vi "Rampfunction (SubVI).vi"(0 "Time":dbl, 1 "Ramp activate":bool, 5 "Ramp td [s]":dbl=1.0, 7 "Ramp tr [s]":dbl=2.0, 9 "Ramp t_ramp [s]":dbl=20.0, 11 "Ramp ymax":dbl=3.5, 12 "Direction":bool) -> (4 "y":dbl, 6 "ramp time":dbl, 8 "Ramp array":dbl[][](array[numeric]), 10 "Ramp active":bool, 15 "Ramp done":bool)   [LabVIEW 2017]
uses:
  <vilib>/gmath/NI_Gmath.lvlib
panel:
  out "y array":dbl[](array[numeric])
  out "time array":dbl[](array[numeric])
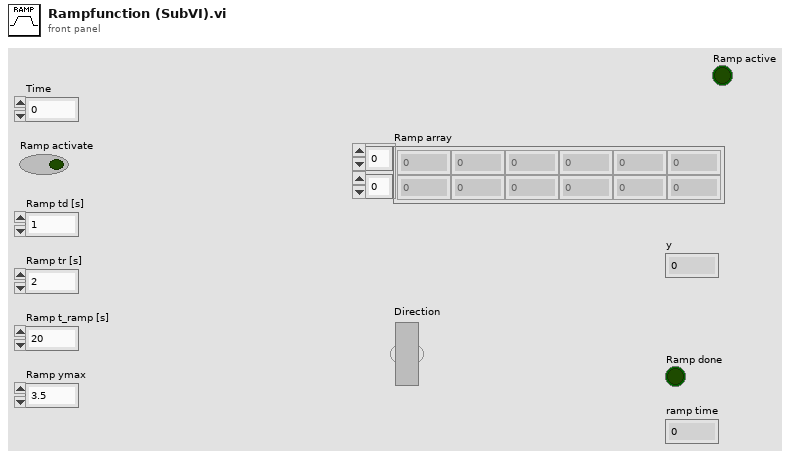
[diagram p1: front panel]
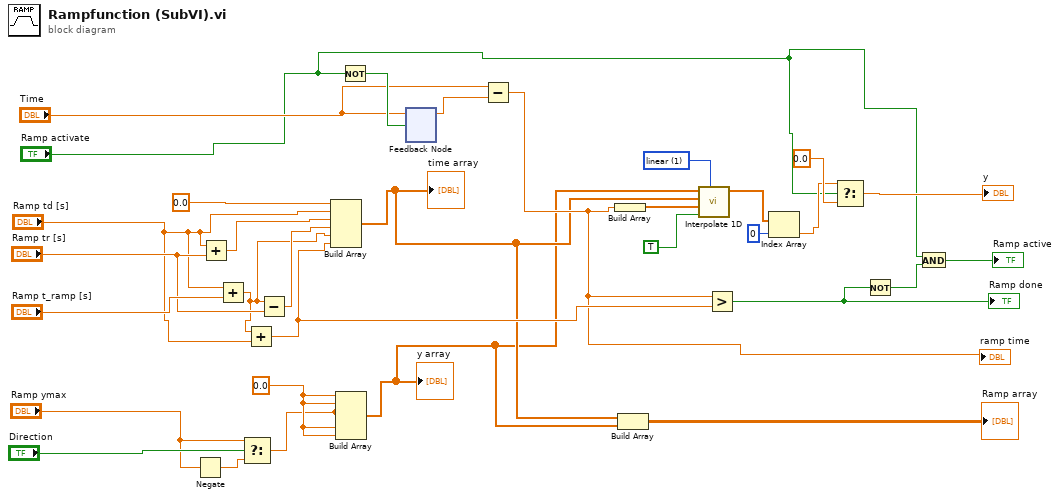
[diagram p0: block diagram]
diagram:
  w27 = 1 items=["nearest", "linear", "spline", "cubic Hermite", "Lagrange"] ("method")
  w13 = 0.0 ("element")
  n1 = Negate(x="Ramp ymax") -> (-x=w3:dbl)
  n2 = Add(x="Ramp td [s]", y="Ramp tr [s]") -> (x+y=w19:dbl)
  n3 = Add(x="Ramp td [s]", y="Ramp t_ramp [s]") -> (x+y=w15:dbl)
  n4 = Select(t="Ramp ymax", s="Direction", f=w3) -> (s? t:f=w1:dbl)
  n5 = Add(x=w15, y="Ramp td [s]") -> (x+y=w23:dbl)
  n6 = Subtract(x=w15, y="Ramp tr [s]") -> (x-y=w16:dbl)
  n7 = Build Array(0.0 ("element"), "Ramp td [s]", w19, w16, w15, w23) -> (w11:dbl[])
  "time array" <- w11
  n8 = Build Array(w13, w13, w1, w1, w13, w13) -> (w10:dbl[])
  "y array" <- w10
  n9 = Not(x="Ramp activate") -> (.not. x?=w30:bool)
  n10 = feedback #1() -> (w29:dbl)  [unwired: 1 in]
  n11 = feedback-in #1("Time", w30) -> ()
  n12 = Subtract(x="Time", y=w29) -> (x-y=w21:dbl)
  "ramp time" <- w21
  n13 = Build Array(w21) -> (w28:dbl[])
  n14 = Build Array(w11, w10) -> (→"Ramp array":dbl[][])
  n15 = call <vilib>:"Interpolate 1D.vi"("method"=w27, "X is monotonic"=TRUE, "xi"=w28, "X"=w11, "Y"=w10) -> ("yi"=w25:dbl[])  [unwired: 4 in, 2 out]
  n16 = Greater?(x=w21, y=w23) -> (0:w6:bool)
  "Ramp done" <- w6
  n17 = Index Array(array=w25, index=0) -> (element=w31:dbl)
  n18 = Select(t=w31, s="Ramp activate", f=0.0) -> (s? t:f=→"y":dbl)
  n19 = Not(x=w6) -> (.not. x?=w7:bool)
  n20 = And(x="Ramp activate", y=w7) -> (x .and. y?=→"Ramp active":bool)
